vi "calibrateEncoder.vi"() -> ()   [LabVIEW 2017]
panel:
  in  "Stop Button":bool
  out "Counter Value":i32
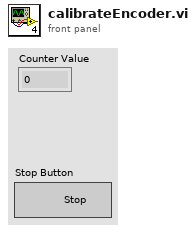
[diagram p1: front panel]
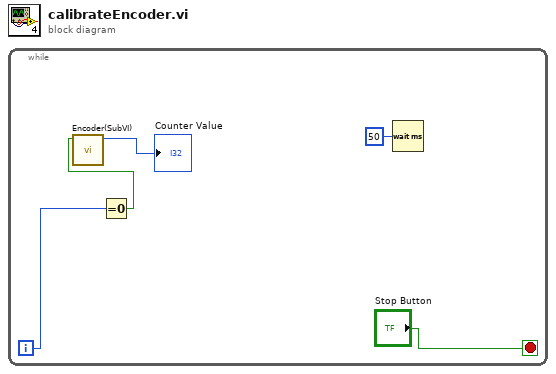
[diagram p0: block diagram]
diagram:
  n1 = while {
    i -> [w2]
    stop <- "Stop Button" stop-if-true
    n2 = Equal To 0?(x=w2) -> (x = 0?=w1:bool)
    n3 = call "Encoder(SubVI).vi"("Reset Counter"=w1) -> ("Counter Value"=→"Counter Value":i32)  [unwired: 9 in, 1 out]
    n4 = Wait (ms)(milliseconds to wait=u32 50) -> ()  [unwired: 1 out]
  }
